vi "MtAtElectrometer_getEvent_settingsAppliedSerConf.vi"(8 "error in (no error)":errorcluster, 11 "logevent_settingsAppliedSerConf_Ctl":T1) -> (0 "error out":errorcluster, 2 "function return":i32, 3 "logevent_settingsAppliedSerConf_Ctl out":T1)   [LabVIEW 2016, in "SALLV_MtAtElectrometer.lvlib"]
doc: "int MtAtElectrometer_shm_getEvent_settingsAppliedSerConfLV(MtAtElectrometer_logevent_settingsAppliedSerConfLV *logevent_settingsAppliedSerConf_Ctl );"
uses:
  SALLV_MtAtElectrometer.lvlib
  DataTypes/logevent_settingsAppliedSerConf.ctl
  ts_sal/test/MtAtElectrometer/labview/SALLV_MtAtElectrometer.so
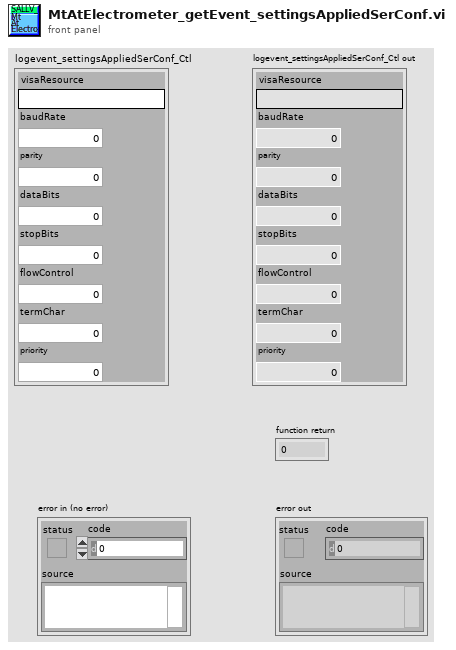
[diagram p1: front panel]
types:
  T1 = typedef "SALLV_MtAtElectrometer.lvlib/logevent_settingsAppliedSerConf.ctl" = cluster{"visaResource":string, "baudRate":i32, "parity":i32, "dataBits":i32, "stopBits":i32, "flowControl":i32, "termChar":i32, "priority":i32}
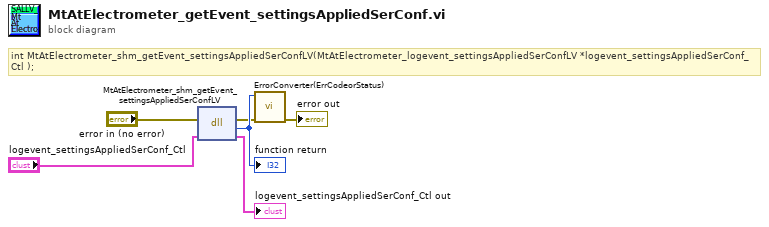
[diagram p0: block diagram]
diagram:
  # "int MtAtElectrometer_shm_getEvent_settingsAppliedSerConfLV(MtAtElectrometer_logevent_settingsAppliedSerConfLV *logevent_settingsAppliedSerConf_Ctl );"
  n1 = dll-call lib="home/andres/ts_sal/test/MtAtElectrometer/labview/SALLV_MtAtElectrometer.*" fn="MtAtElectrometer_shm_getEvent_settingsAppliedSerConfLV"(error in="error in (no error)", "logevent_settingsAppliedSerConf_Ctl"="logevent_settingsAppliedSerConf_Ctl") -> (error out=w2:errorcluster, w6:i32, "logevent_settingsAppliedSerConf_Ctl"=→"logevent_settingsAppliedSerConf_Ctl out":T1)  [unwired: 2 in, 1 out]
  "function return" <- w6
  n2 = call "ErrorConverter(ErrCodeorStatus).vi"("error in (no error)"=w2, "error code"=w6) -> ("error out"=→"error out":errorcluster)  [unwired: 9 in]
